vi "getCorners.vi"(8 "error in (no error)":errorcluster, 11 "StationKeeping in":refnum<class "StationKeeping.lvclass">) -> (0 "error out":errorcluster, 1 "Buoy SW":T1 {"North" format="%#_10f"; "East" format="%#_8f"}, 2 "Buoy NE":T1 {"North" format="%#_10f"; "East" format="%#_8f"}, 3 "StationKeeping out":refnum<class "StationKeeping.lvclass">, 4 "Buoy SE":T1 {"North" format="%#_10f"; "East" format="%#_8f"}, 5 "Buoy NW":T1 {"North" format="%#_10f"; "East" format="%#_8f"})   [LabVIEW 2011, in "StationKeeping.lvclass"]
doc: "Returns the four corners of the station."
uses:
  StationKeeping.lvclass
  2 Typedefs/UTM Location.ctl
  StationKeeping.lvclass/StationKeeping.ctl
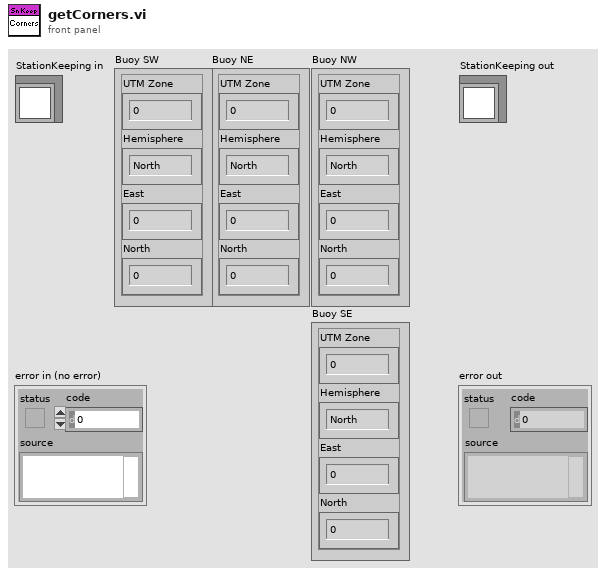
[diagram p1: front panel]
types:
  T1 = typedef "UTM Location.ctl" = cluster{"UTM Zone":dbl, "Hemisphere":enum16{"North", "South"}, "East":dbl, "North":dbl}
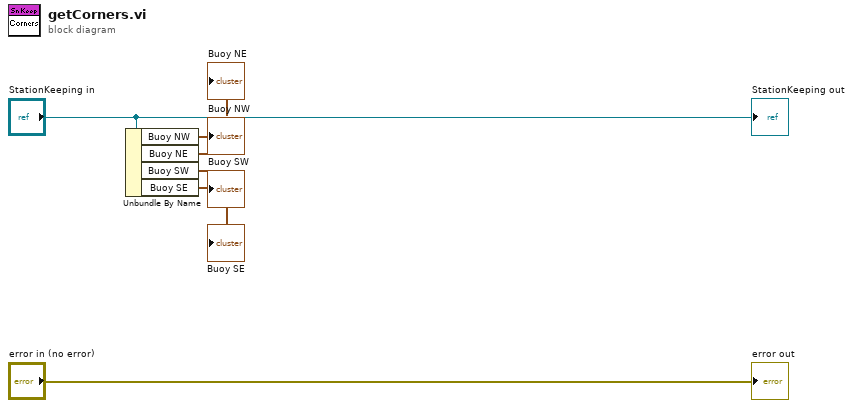
[diagram p0: block diagram]
diagram:
  n1 = Unbundle By Name("StationKeeping in") -> ("Buoy NW"=→"Buoy NW":T1, "Buoy NE"=→"Buoy NE":T1, "Buoy SW"=→"Buoy SW":T1, "Buoy SE"=→"Buoy SE":T1)
  "error out" <- "error in (no error)"
  "StationKeeping out" <- "StationKeeping in"
